vi "New Error File Dialog.vi"(8 "error in (no error)":errorcluster, 11 "project path in":path) -> (0 "error out":errorcluster, 1 "canceled?":bool, 2 "file path":path, 3 "project path dup":path)   [LabVIEW 2017]
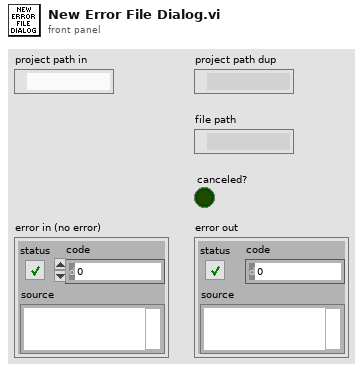
[diagram p1: front panel]
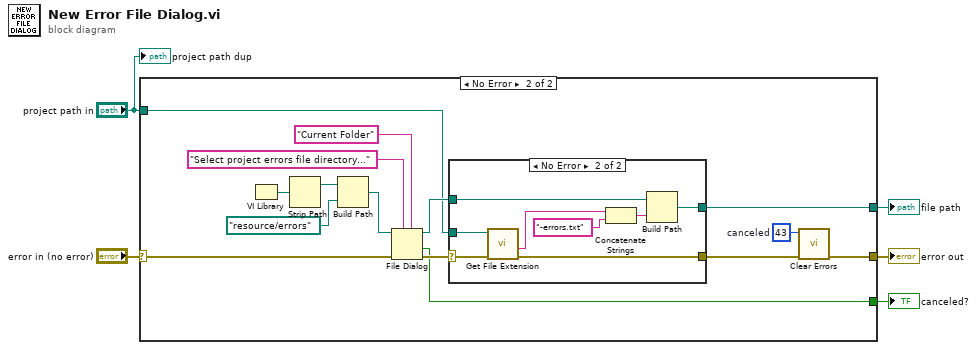
[diagram p0: block diagram]
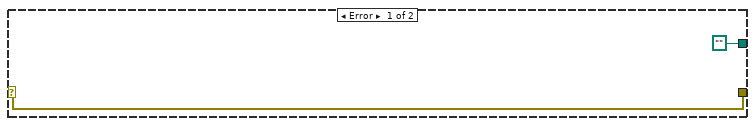
[diagram p2: hidden frame]
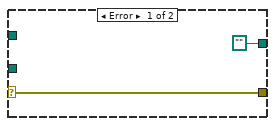
[diagram p3: hidden frame]
diagram:
  n1 = case shown="No Error" "error in (no error)" {
    selector: "error in (no error)" -> [w7 w8]
    tunnel: [path "" w13] -> w5
    tunnel: [_ w12] -> w4
    tunnel: "project path in" -> [_ w10]
    tunnel: [w7 w9] -> w1
    frame Error {
    }
    frame No Error {
      w16 = 43  # canceled
      n2 = VI Library() -> (path=w22:path)
      n3 = Strip Path(path=w22) -> (stripped path=w21:path)  [unwired: 1 out]
      n4 = Build Path(base path=w21, name or relative path=path "resource/errors") -> (appended path=w19:path)
      n5 = File Dialog(5:"Current Folder" ("button label"), 7:"Select project errors file directory..." ("prompt"), 8:w8, 11:w19) -> (0:w14:errorcluster, 1:w12:bool, 3:w15:path)  [unwired: 3 in, 1 out]
      n6 = case shown="No Error" w14 {
        selector: w14 -> [w24 w28]
        tunnel: w15 -> [_ w25]
        tunnel: [w24 w29] -> w11
        tunnel: w10 -> [_ w27]
        tunnel: [path "" w26] -> w13
        frame Error {
        }
        frame No Error {
          n7 = call <vilib>:"Get File Extension.vi"("error in (no error)"=w28, "file"=w27) -> ("error out"=w29:errorcluster, "filename without extension"=w32:string)  [unwired: 5 in, 3 out]
          n8 = Concatenate Strings(w32, "-errors.txt" ("string")) -> (w31:string)
          n9 = Build Path(base path=w25, name or relative path=w31) -> (appended path=w26:path)
        }
      }
      n10 = call <vilib>:"Clear Errors.vi"("error in (no error)"=w11, "specific error code to clear (0: all)"=w16) -> ("error out"=w9:errorcluster)  [unwired: 4 in, 1 out]
    }
  }
  "file path" <- w5
  "canceled?" <- w4
  "error out" <- w1
  "project path dup" <- "project path in"
